vi "Save Recall Instrument Settings.vi"(8 "error in (no error)":errorcluster, 9 "Memory Location (0)":dbl min=0.0 max=9.0 format="%#_0f", 10 "Save Recall Settings (0:Save)":i32(ring) items=["Save", "Recall"], 11 "VISA resource name":refnum<visa-resource-name>) -> (0 "error out":errorcluster, 3 "VISA resource name out":refnum<visa-resource-name>)   [LabVIEW 2020, in "BK Precision 911X Series.lvlib"]
doc: "Saves or recalls instrument settings to or from a specified memory location."
uses:
  BK Precision 911X Series.lvlib
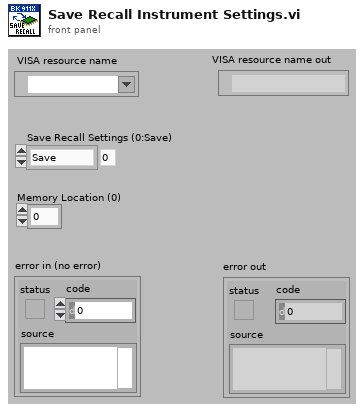
[diagram p1: front panel]
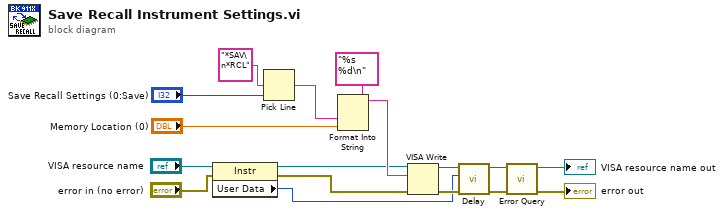
[diagram p0: block diagram]
diagram:
  n1 = property class="Instr"(reference="VISA resource name", error in="error in (no error)") -> (reference out=w3:refnum<visa-resource-name>, error out=w1:errorcluster, "User Data"=w2:u32)
  n2 = Pick Line(multi-line string="*SAV\n*RCL", line index="Save Recall Settings (0:Save)") -> (output string=w14:string)  [unwired: 1 in]
  n3 = Format Into String(format string="%s %d\n", w14, "Memory Location (0)") -> (resulting string=w11:string)  [unwired: 2 in, 1 out]
  n4 = VISA Write(VISA resource name=w3, write buffer=w11, error in (no error)=w1) -> (VISA resource name out=w9:refnum<visa-resource-name>, error out=w8:errorcluster)  [unwired: 1 out]
  n5 = call "Delay.vi"("error in (no error)"=w8, "Delay Time (0 ms)"=w2, "VISA resource name"=w9) -> ("error out"=w6:errorcluster, "VISA resource name out"=w7:refnum<visa-resource-name>)  [unwired: 7 in]
  n6 = call "Error Query.vi"("error in (no error)"=w6, "VISA resource name"=w7) -> ("error out"=→"error out":errorcluster, "VISA resource name out"=→"VISA resource name out":refnum<visa-resource-name>)  [unwired: 6 in, 2 out]
